vi "SPI Sensor Processing.vi"(11 "stop":bool) -> ()   [LabVIEW 2014]
uses:
  <vilib>/rvi/interface/nirviOpenFPGA/nirviOpenFPGA.xnode
  FPGA/Sensor Library/FPGA.vi
  SPI/Controls/FPGA Reference.ctl
  Global Data.vi
  <vilib>/rvi/interface/nirviCloseFPGA/nirviCloseFPGA.xnode
  <vilib>/FPGAPlugInAG/sbRIO-9626/niLvFpga_Close_sbRIO-9626.vi
  FPGA Telemetry.ctl
  MC State Machine.lvsc/State.ctl
  MC State Machine.lvsc
  Reason for Shutdown.ctl
  AIR Status.ctl
  Shutdown State Machine.lvsc/State.ctl
  Shutdown State Machine.lvsc
  Vehicle Status/Subsystem Status.ctl
  Dash LED Status.ctl
  FPGA Loads and Shutdown.ctl
  FPGA Bitfiles/FormulaElectric2_FPGATarget_FPGA_8a5J0mMac2U.lvbitx
  <vilib>/FPGAPlugInAG/sbRIO-9626/niLvFpga_Open_sbRIO-9626.vi
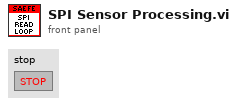
[diagram p1: front panel]
types:
  T1 = typedef "FPGA Reference.ctl" = refnum<k20>
  T2 = typedef "FPGA Telemetry.ctl" = cluster{"sbRIO":cluster{"Supply Voltage (V)":fxp<+/-,25,6>, "FPGA LED":bool, "Chassis Temperature":fxp<+/-,16,9>}, "Throttles":cluster{"Throttles Consistent?":bool, "Throttles In Range?":bool, "Average Throttle (%)":fxp<+/-,29,18>, "Throttle 2 (V)":fxp<+/-,24,5>, "Throttle 2 (%)":fxp<+/-,27,18>, "Throttle 1 (V)":fxp<+/-,24,5>, "Throttle 1 (%)":fxp<+/-,27,18>, "Throttle 2 Max":fxp<+,16,4>, "Throttle 2 Min":fxp<+,16,4>, "Throttle 1 Max":fxp<+,16,4>, "Throttle 1 Min":fxp<+,16,4>}, "Loads & Shutdown":T3, "Motor Controller":cluster{"Motor Controller Dash Switch":bool, "Motor Controller Enable":bool}, "Sensors":cluster{"RL Tick Period":u32, "RR Tick Period":u32, "FR Tick Period":u32, "FL Tick Period":u32, "RR Shock (V)":fxp<+/-,24,5>, "RL Shock (V)":fxp<+/-,24,5>, "FR Shock (V)":fxp<+/-,24,5>, "FL Shock (V)":fxp<+/-,24,5>, "RR Stopped":bool, "RL Stopped":bool, "FR Stopped":bool, "FL Stopped":bool, "Steering Wheel Middle":fxp<+/-,26,5>, "Steering Wheel Angle (degrees)":fxp<+/-,31,13>, "High Current OK?":bool, "Low Current OK?":bool, "Rear BPS OK?":bool, "Front BPS OK?":bool, "Rear BP (psi)":fxp<+/-,27,16>, "Front BP (psi)":fxp<+/-,27,16>, "High Current (A)":fxp<+/-,24,15>, "Low Current (A)":fxp<+/-,24,15>, "RR State":bool, "RL State":bool, "FR State":bool, "FL State":bool}, "CPU Load":cluster{"Total (%)":dbl, "Time Critical (%)":dbl, "Timed Structures (%)":dbl, "High (%)":dbl, "Above Normal (%)":dbl, "Normal (%)":dbl, "Background (%)":dbl, "Idle (%)":dbl, "ISR (%)":dbl}, "Vehicle Status":cluster{"BMS Status":T5, "MC Status":T5, "Shutdown Status":T5, "sbRIO Status":T5, "Vehicle Status":T5, "Shutdown State":T6, "AIR Status":T7, "Remote Return to Pits":bool, "Reason for Shutdown":T8, "MC State Machine Status":T9}}
  T3 = typedef "FPGA Loads and Shutdown.ctl" = cluster{"RTDS Enable":bool, "TSMS In Status":bool, "Positive AIR Enable":bool, "cRIO Shutdown 2":bool, "cRIO Shutdown 1":bool, "TSMS Out Status":bool, "Coolant Pump":bool, "BMS OK":bool, "IMD In":bool, "BSPD In":bool, "Brake Light Out":bool, "Green LED":T4, "Yellow LED":T4, "Red LED":T4}
  T4 = typedef "Dash LED Status.ctl" = enum16{"Off", "Flashing", "On"}
  T5 = typedef "Subsystem Status.ctl" = enum16{"Okay", "Short Warning", "Long Warning", "Return to Pits", "Error", "Danger"}
  T6 = typedef "Shutdown State Machine.lvsc/State.ctl" = enum16{"NI.SC.Initial", "NI.SC.History", "NI.SC.ShallowHistory", "NI.SC.Terminal", "Coolant Pump Started/AIR's On", "AIRs On", "Precharge", "TSMS Off"}
  T7 = typedef "AIR Status.ctl" = enum16{"Off", "Precharge", "On"}
  T8 = typedef "Reason for Shutdown.ctl" = enum16{"None", "BMS", "Shutdown", "sbRIO", "MC", "Remote"}
  T9 = typedef "MC State Machine.lvsc/State.ctl" = enum16{"NI.SC.Initial", "NI.SC.History", "NI.SC.ShallowHistory", "NI.SC.Terminal", "Let Current Drop then Disable AIR's", "Enabled", "Disabled"}
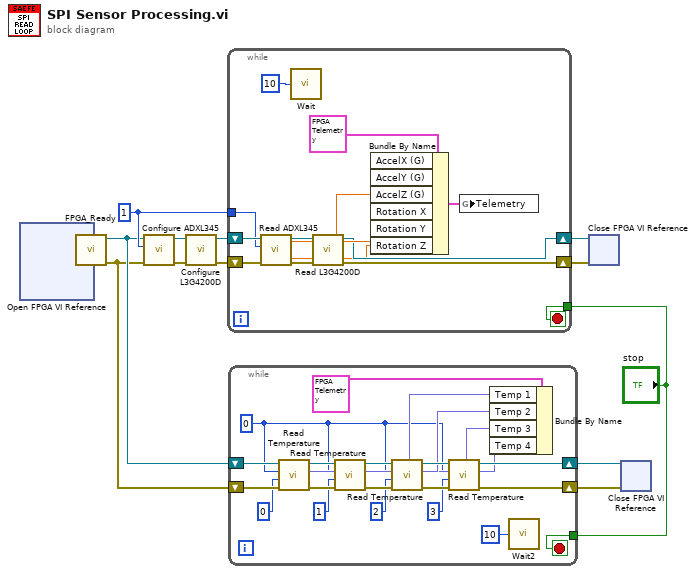
[diagram p0: block diagram]
diagram:
  w12 = i8 1 ("Port")
  n1 = xnode "Open FPGA VI Reference"() -> ("FPGA VI Reference Out"=w14:T1, "error out"=w13:errorcluster)  [unwired: 2 in]
  n2 = call "FPGA_Ready.vi"("Error In"=w13, "FPGA VI Reference In"=w14) -> ("Error Out"=w4:errorcluster, "FPGA VI Reference Out"=w5:T1)  [unwired: 7 in]
  n3 = call "Configure ADXL345.vi"("error in"=w4, "Port"=w12, "FPGA VI Reference"=w5) -> ("error out"=w8:errorcluster, "FPGA VI Reference Out"=w9:T1)  [unwired: 7 in]
  n4 = call "Configure L3G4200D.vi"("error in"=w8, "FPGA VI Reference"=w9) -> ("error out"=w10:errorcluster, "FPGA VI Reference Out"=w11:T1)  [unwired: 8 in]
  n5 = while {
    tunnel: w12 -> [w29]
    shift-right: [w22] -> w6
    shift-left: w10 -> [w30]
    shift-right: [w23] -> w7
    shift-left: w11 -> [w31]
    tunnel: "stop" -> [w15]
    stop <- w15 stop-if-true
    n6 = call "Read ADXL345.vi"("Error In"=w30, "Port"=w29, "FPGA VI Reference In"=w31) -> ("error out"=w24:errorcluster, "FPGA VI Reference Out"=w25:T1, "Y"=w27:dbl, "Z"=w26:dbl, "X"=w28:dbl)  [unwired: 4 in]
    n7 = call "Wait"("Count(mSec)"=u32 10) -> ()  [unwired: 1 out]
    n8 = call "Read L3G4200D.vi"("Error In"=w24, "FPGA VI Reference In"=w25) -> ("error out"=w22:errorcluster, "FPGA VI Reference Out"=w23:T1, "Z Rotation Rate (mdps)"=w19:dbl, "Y Rotation Rate (mdps)"=w20:dbl, "X Rotation Rate (mdps)"=w21:dbl)  [unwired: 5 in]
    n9 = Bundle By Name(cluster=T2 {"sbRIO"={"Supply Voltage (V)"=0.0, "FPGA LED"=FALSE, "Chassis Temperature"=0.0}, "Throttles"={"Throttles Consistent?"=FALSE, "Throttles In Range?"=FALSE, "Average Throttle (%)"=185.44775390625, "Throttle 2 (V)"=0.0, "Throttle 2 (%)"=-866.732421875, "Throttle 1 (V)"=15.999998092651367, "Throttle 1 (%)"=0.34765625, "Throttle 2 Max"=0.0, "Throttle 2 Min"=0.0, "Throttle 1 Max"=0.0, "Throttle 1 Min"=0.0}, "Loads & Shutdown"={"RTDS Enable"=FALSE, "TSMS In Status"=FALSE, "Positive AIR Enable"=FALSE, "cRIO Shutdown 2"=TRUE, "cRIO Shutdown 1"=TRUE, "TSMS Out Status"=FALSE, "Coolant Pump"=FALSE, "BMS OK"=FALSE, "IMD In"=FALSE, "BSPD In"=FALSE, "Brake Light Out"=TRUE, "Green LED"=enum."On", "Yellow LED"=enum."Off", "Red LED"=enum."Off"}, "Motor Controller"={"Motor Controller Dash Switch"=TRUE, "Motor Controller Enable"=TRUE}, "Sensors"={"RL Tick Period"=0, "RR Tick Period"=0, "FR Tick Period"=0, "FL Tick Period"=0, "RR Shock (V)"=0.0, "RL Shock (V)"=0.0, "FR Shock (V)"=0.0, "FL Shock (V)"=0.0, "RR Stopped"=TRUE, "RL Stopped"=TRUE, "FR Stopped"=TRUE, "FL Stopped"=TRUE, "Steering Wheel Middle"=0.0, "Steering Wheel Angle (degrees)"=0.0, "High Current OK?"=FALSE, "Low Current OK?"=FALSE, "Rear BPS OK?"=TRUE, "Front BPS OK?"=TRUE, "Rear BP (psi)"=0.0, "Front BP (psi)"=0.0, "High Current (A)"=0.0, "Low Current (A)"=0.0, "RR State"=FALSE, "RL State"=FALSE, "FR State"=FALSE, "FL State"=FALSE}, "CPU Load"={"Total (%)"=0.0, "Time Critical (%)"=0.0, "Timed Structures (%)"=0.0, "High (%)"=0.0, "Above Normal (%)"=1.0, "Normal (%)"=1.0, "Background (%)"=0.0, "Idle (%)"=0.0, "ISR (%)"=0.0}, "Vehicle Status"={"BMS Status"=enum."Okay", "MC Status"=enum."Okay", "Shutdown Status"=enum."Okay", "sbRIO Status"=enum."Okay", "Vehicle Status"=enum."Okay", "Shutdown State"=enum."NI.SC.Initial", "AIR Status"=enum."Off", "Remote Return to Pits"=FALSE, "Reason for Shutdown"=enum."None", "MC State Machine Status"=enum."NI.SC.Initial"}} ("Telemetry"), "AccelX (G)"=w28, "AccelY (G)"=w27, "AccelZ (G)"=w26, "Rotation X"=w21, "Rotation Y"=w20, "Rotation Z"=w19) -> (w16:T2)
    n10 = global write "Global Data.vi" "Telemetry"(w16) -> ()
  }
  n11 = while {
    shift-right: [w42] -> w3
    shift-left: w5 -> [w53]
    shift-right: [w43] -> w2
    shift-left: w4 -> [w52]
    tunnel: "stop" -> [w51]
    stop <- w51 stop-if-true
    w36 = i8 0 ("Port")
    n12 = call "Read Temperature.vi"("Error In"=w52, "Thermocouple #"=u8 0, "Port"=w36, "FPGA VI Reference In"=w53) -> ("error out"=w46:errorcluster, "Temperature Out (C)"=w40:fxp<+,12,10>, "FPGA VI Reference Out"=w49:T1)  [unwired: 5 in]
    n13 = call "Read Temperature.vi"("Error In"=w46, "Thermocouple #"=u8 1, "Port"=w36, "FPGA VI Reference In"=w49) -> ("error out"=w45:errorcluster, "Temperature Out (C)"=w39:fxp<+,12,10>, "FPGA VI Reference Out"=w48:T1)  [unwired: 5 in]
    n14 = call "Read Temperature.vi"("Error In"=w45, "Thermocouple #"=u8 2, "Port"=w36, "FPGA VI Reference In"=w48) -> ("error out"=w44:errorcluster, "Temperature Out (C)"=w38:fxp<+,12,10>, "FPGA VI Reference Out"=w47:T1)  [unwired: 5 in]
    n15 = call "Read Temperature.vi"("Error In"=w44, "Thermocouple #"=u8 3, "Port"=w36, "FPGA VI Reference In"=w47) -> ("error out"=w43:errorcluster, "Temperature Out (C)"=w37:fxp<+,12,10>, "FPGA VI Reference Out"=w42:T1)  [unwired: 5 in]
    n16 = Bundle By Name(cluster=T2 {"sbRIO"={"Supply Voltage (V)"=0.0, "FPGA LED"=FALSE, "Chassis Temperature"=0.0}, "Throttles"={"Throttles Consistent?"=FALSE, "Throttles In Range?"=FALSE, "Average Throttle (%)"=185.44775390625, "Throttle 2 (V)"=0.0, "Throttle 2 (%)"=-866.732421875, "Throttle 1 (V)"=15.999998092651367, "Throttle 1 (%)"=0.34765625, "Throttle 2 Max"=0.0, "Throttle 2 Min"=0.0, "Throttle 1 Max"=0.0, "Throttle 1 Min"=0.0}, "Loads & Shutdown"={"RTDS Enable"=FALSE, "TSMS In Status"=FALSE, "Positive AIR Enable"=FALSE, "cRIO Shutdown 2"=TRUE, "cRIO Shutdown 1"=TRUE, "TSMS Out Status"=FALSE, "Coolant Pump"=FALSE, "BMS OK"=FALSE, "IMD In"=FALSE, "BSPD In"=FALSE, "Brake Light Out"=TRUE, "Green LED"=enum."On", "Yellow LED"=enum."Off", "Red LED"=enum."Off"}, "Motor Controller"={"Motor Controller Dash Switch"=TRUE, "Motor Controller Enable"=TRUE}, "Sensors"={"RL Tick Period"=0, "RR Tick Period"=0, "FR Tick Period"=0, "FL Tick Period"=0, "RR Shock (V)"=0.0, "RL Shock (V)"=0.0, "FR Shock (V)"=0.0, "FL Shock (V)"=0.0, "RR Stopped"=TRUE, "RL Stopped"=TRUE, "FR Stopped"=TRUE, "FL Stopped"=TRUE, "Steering Wheel Middle"=0.0, "Steering Wheel Angle (degrees)"=0.0, "High Current OK?"=FALSE, "Low Current OK?"=FALSE, "Rear BPS OK?"=TRUE, "Front BPS OK?"=TRUE, "Rear BP (psi)"=0.0, "Front BP (psi)"=0.0, "High Current (A)"=0.0, "Low Current (A)"=0.0, "RR State"=FALSE, "RL State"=FALSE, "FR State"=FALSE, "FL State"=FALSE}, "CPU Load"={"Total (%)"=0.0, "Time Critical (%)"=0.0, "Timed Structures (%)"=0.0, "High (%)"=0.0, "Above Normal (%)"=1.0, "Normal (%)"=1.0, "Background (%)"=0.0, "Idle (%)"=0.0, "ISR (%)"=0.0}, "Vehicle Status"={"BMS Status"=enum."Okay", "MC Status"=enum."Okay", "Shutdown Status"=enum."Okay", "sbRIO Status"=enum."Okay", "Vehicle Status"=enum."Okay", "Shutdown State"=enum."NI.SC.Initial", "AIR Status"=enum."Off", "Remote Return to Pits"=FALSE, "Reason for Shutdown"=enum."None", "MC State Machine Status"=enum."NI.SC.Initial"}} ("Telemetry"), "Temp 1"=w40, "Temp 2"=w39, "Temp 3"=w38, "Temp 4"=w37) -> ()  [unwired: 1 out]
    n17 = call "Wait2"("Count(mSec)"=u32 10) -> ()  [unwired: 1 out]
  }
  n18 = xnode "Close FPGA VI Reference"("FPGA VI Reference In"=w7, "error in"=w6) -> ()  [unwired: 1 out]
  n19 = xnode "Close FPGA VI Reference"("FPGA VI Reference In"=w3, "error in"=w2) -> ()  [unwired: 1 out]
